vi "Profile Test.vi"() -> ()   [LabVIEW 2018]
panel:
  in  "Driver Selection":u16(ring) items=["Amelia", "Ashley"]
  out "Current Deadband":dbl
  out "Driver you are Editing":string
  in  "Recognized Drivers":string[](array[string])
  in  "Deadband":dbl[](array[numeric])
  # "ON DRIVER STATION"
  # "ON ROBOT"
  # "ON ROBOT"
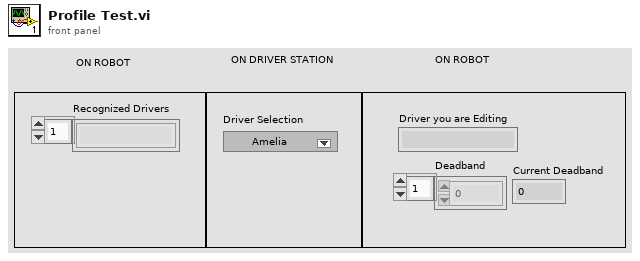
[diagram p1: front panel]
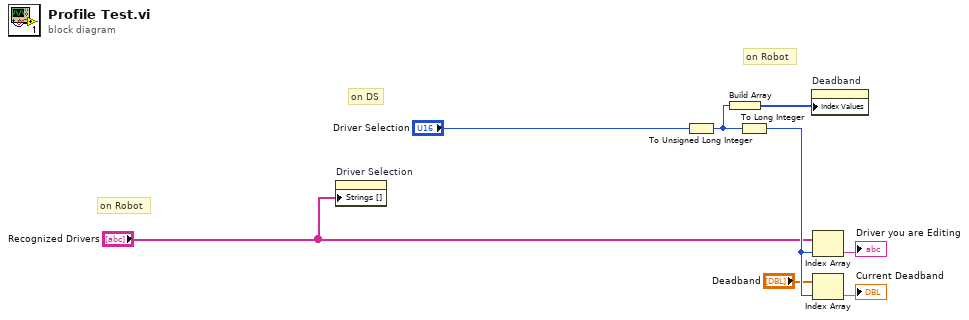
[diagram p0: block diagram]
diagram:
  # "on Robot"
  # "on DS"
  # "on Robot"
  n1 = property on="Driver Selection" class="Ring (strict)"("Strings []"="Recognized Drivers") -> ()  [unwired: 2 in, 2 out]
  n2 = To Unsigned Long Integer(number="Driver Selection") -> (unsigned 32bit integer=w1:u32)
  n3 = Build Array(w1) -> (w7:u32[])
  n4 = To Long Integer(number=w1) -> (32bit integer=w6:i32)
  n5 = property on="Deadband" class="Arr (strict)"("Index Values"=w7) -> ()  [unwired: 2 in, 2 out]
  n6 = Index Array(array="Recognized Drivers", index=w6) -> (element=→"Driver you are Editing":string)
  n7 = Index Array(array="Deadband", index=w6) -> (element=→"Current Deadband":dbl)
